vi "Show Hide Hourglass.vi"(6 "Action":enum16{"Hide", "Show"}(ring), 8 "error in (no error)":errorcluster, 11 "Pic Size":T1={"Width"=70, "Height"=70}) -> (0 "error IO":errorcluster)   [LabVIEW 2020]
uses:
  <vilib>/Utility/miscctls.llb/LVBoundsTypeDef.ctl
panel:
  # "USE THIS IMAGE. Dimensions are 70x70"
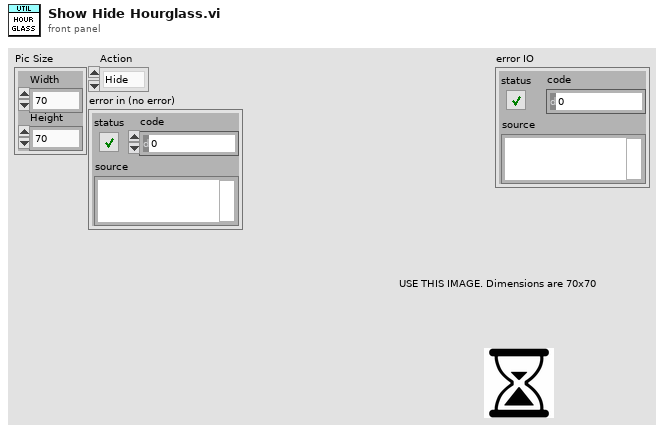
[diagram p1: front panel]
types:
  T1 = typedef "LVBoundsTypeDef.ctl" = cluster{"Width":u32, "Height":u32}
  T2 = enum8{"Enabled", "Disabled", "Disabled and Grayed Out"}[]
  T3 = enum8{"Enabled", "Disabled", "Disabled and Grayed Out"}
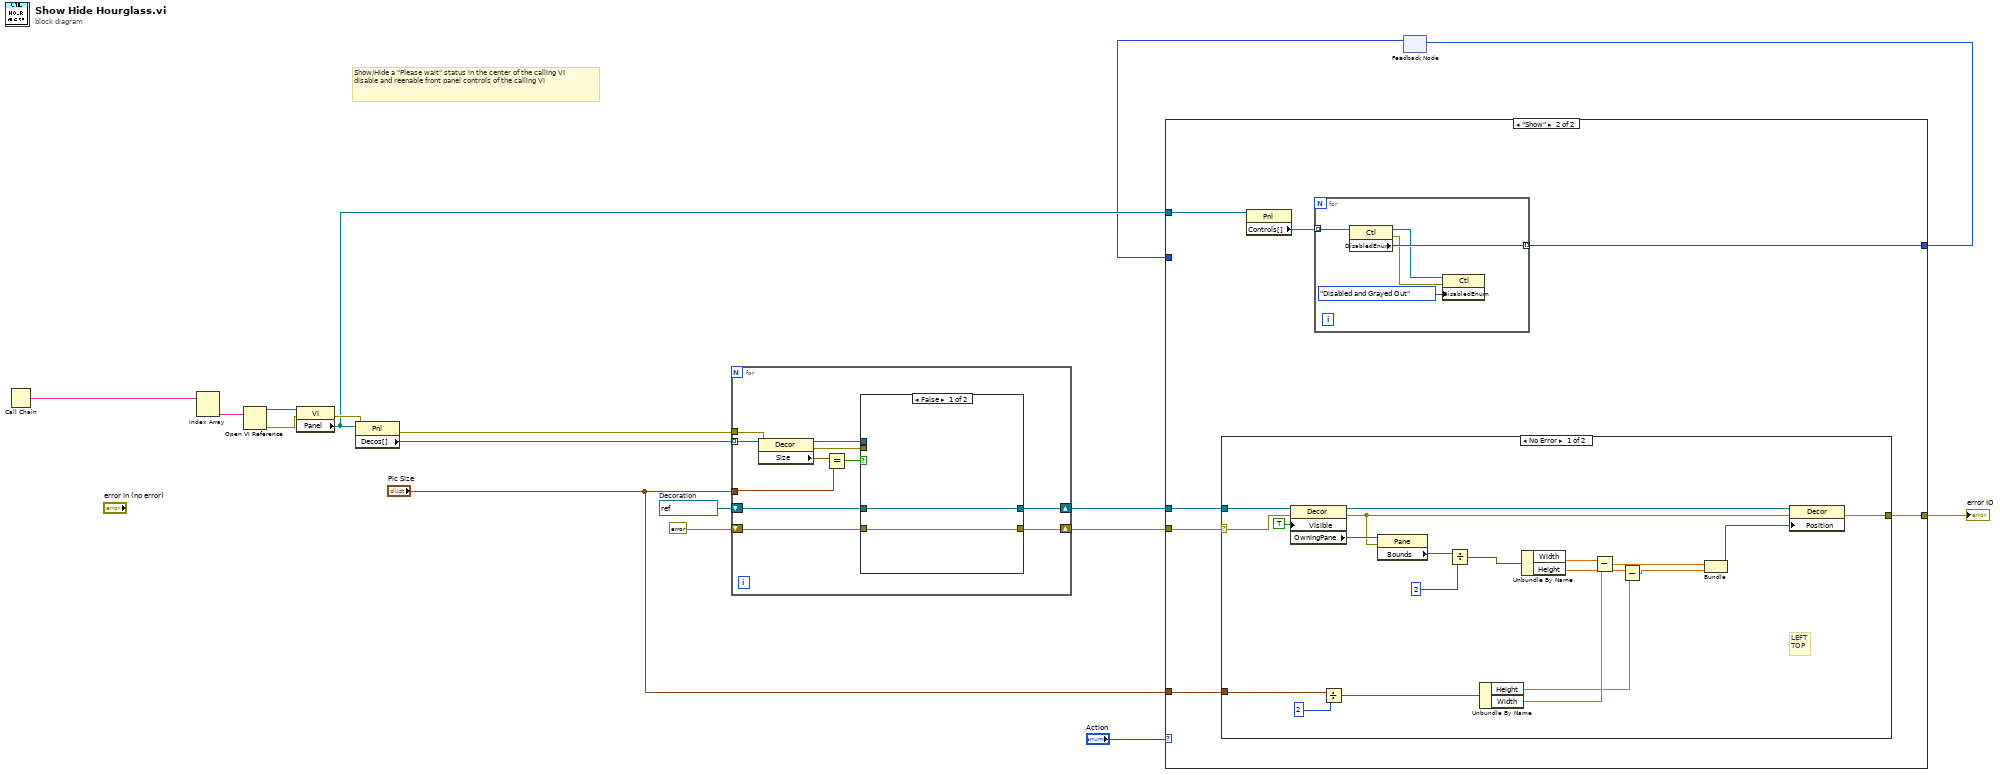
[diagram p0: block diagram]
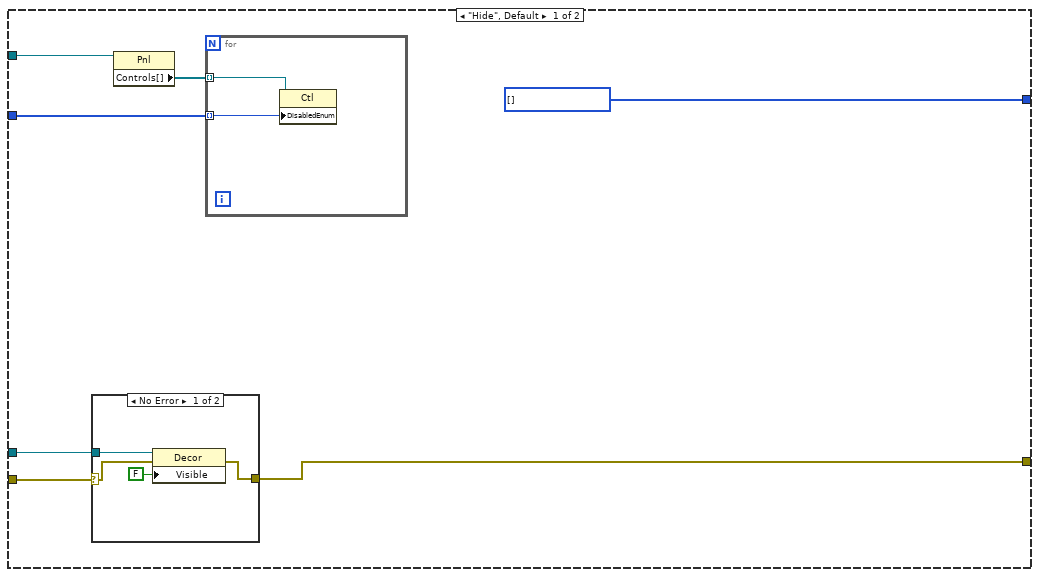
[diagram p2: hidden frame]
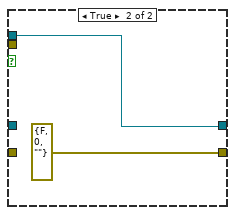
[diagram p5: hidden frame]
diagram:
  w13 = refnum<vi> refnum  # Decoration
  # "Show/Hide a \"Please wait\" status in the center of the calling VI\ndisable and reenable front panel controls of the calling VI"
  n1 = Call Chain() -> (call chain=w17:string[])
  n2 = Index Array(array=w17) -> (element #2=w16:string)  [unwired: 2 in, 1 out]
  n3 = Open VI Reference(vi path=w16) -> (vi reference=w15:refnum<vi>, error out=w10:errorcluster)  [unwired: 5 in]
  n4 = property class="VI"(reference=w15, error in=w10) -> (error out=w11:errorcluster, "Panel"=w4:refnum<vi>)  [unwired: 1 out]
  n5 = property class="Pnl"(reference=w4, error in=w11) -> (error out=w12:errorcluster, "Decos[]"=w14:refnum<vi>[])  [unwired: 1 out]
  n6 = for {
    tunnel: w14 -> [w28] mode=indexing
    tunnel: "Pic Size" -> [w26]
    shift-right: [w22] -> w9
    shift-left: w13 -> [w23]
    tunnel: w12 -> [w20]
    shift-right: [w18] -> w7
    shift-left: errorcluster {"status"=TRUE, "code"=0, "source"="Wait Icon not Found"} ("error out") -> [w19]
    n7 = property class="Decor"(reference=w28, error in=w20) -> (reference out=w24:refnum<vi>, error out=w21:errorcluster, "Size"=w27:T1)
    n8 = Equal?(x=w27, y=w26) -> (x = y?=w25:bool)
    n9 = case shown="False" w25 {
      tunnel: w24 -> [_ w32]
      tunnel: w23 -> [w30 _]
      tunnel: [w30 w32] -> w22
      tunnel: w21 -> [_ _]
      tunnel: w19 -> [w29 _]
      tunnel: [w29 errorcluster {"status"=FALSE, "code"=0, "source"=""} ("error out")] -> w18
      frame False {
      }
      frame True {
      }
    }
  }
  n10 = feedback #1() -> (w2:T2)  [unwired: 1 in]
  n11 = case shown="\"Show\"" "Action" {
    tunnel: w9 -> [w38 w53]
    tunnel: w7 -> [w37 w52]
    tunnel: [w39 w51] -> w5
    tunnel: w4 -> [w35 w49]
    tunnel: [w33 w48] -> w3
    tunnel: w2 -> [w34 _]
    tunnel: "Pic Size" -> [_ w47]
    frame "Hide", Default {
      w33 = T2 [] items=["Enabled", "Disabled", "Disabled and Grayed Out"]
      n12 = case shown="No Error" w37 {
        selector: w37 -> [w43 w46]
        tunnel: w38 -> [w44 _]
        tunnel: [w42 w46] -> w39
        frame No Error {
          n13 = property class="Decor"(reference=w44, error in=w43, "Visible"=FALSE) -> (error out=w42:errorcluster)  [unwired: 1 out]
        }
        frame Error {
        }
      }
      n14 = property class="Pnl"(reference=w35) -> ("Controls[]"=w36:refnum<vi>[])  [unwired: 1 in, 2 out]
      n15 = for {
        tunnel: w36 -> [w41] mode=indexing
        tunnel: w34 -> [w40] mode=indexing
        n16 = property class="Ctl"(reference=w41, "DisabledEnum"=w40) -> ()  [unwired: 1 in, 2 out]
      }
    }
    frame "Show" {
      n17 = case shown="No Error" w52 {
        selector: w52 -> [w76 w79]
        tunnel: w53 -> [w78 _]
        tunnel: [w69 w79] -> w51
        tunnel: w47 -> [w74 _]
        frame No Error {
          # "LEFT\nTOP"
          n18 = property class="Decor"(reference=w78, error in=w76, "Visible"=TRUE) -> (reference out=w71:refnum<vi>, error out=w70:errorcluster, "OwningPane"=w75:refnum<vi>)
          n19 = Divide(x=w74, y=i16 2) -> (x/y=w72:cluster{"Width":dbl, "Height":dbl})
          n20 = property class="Pane"(reference=w75, error in=w70) -> ("Bounds"=w68:T1)  [unwired: 2 out]
          n21 = Divide(x=w68, y=2) -> (x/y=w66:cluster{"Width":dbl, "Height":dbl})
          n22 = Unbundle By Name(w72) -> ("Height"=w62:dbl, "Width"=w64:dbl)
          n23 = Unbundle By Name(w66) -> ("Width"=w65:dbl, "Height"=w63:dbl)
          n24 = Subtract(x=w65, y=w64) -> (x-y=w61:dbl)
          n25 = Subtract(x=w63, y=w62) -> (x-y=w60:dbl)
          n26 = Bundle(w61, w60) -> (w59:cluster{dbl, dbl})  [unwired: 1 in]
          n27 = property class="Decor"(reference=w71, error in=w70, "Position"=w59) -> (error out=w69:errorcluster)  [unwired: 1 out]
        }
        frame Error {
        }
      }
      n28 = property class="Pnl"(reference=w49) -> ("Controls[]"=w50:refnum<vi>[])  [unwired: 1 in, 2 out]
      n29 = for {
        tunnel: w50 -> [w58] mode=indexing
        tunnel: [w57] -> w48 mode=indexing
        n30 = property class="Ctl"(reference=w58) -> (reference out=w56:refnum<vi>, error out=w55:errorcluster, "DisabledEnum"=w57:T3)  [unwired: 1 in]
        n31 = property class="Ctl"(reference=w56, error in=w55, "DisabledEnum"=T3."Disabled and Grayed Out" ("Disabled")) -> ()  [unwired: 2 out]
      }
    }
  }
  "error IO" <- w5
  n32 = feedback-in #1(w3) -> ()
